vi "sendOutputData.vi"(8 "error in (no error)":errorcluster, 11 "Model in":refnum<class "Model.lvclass">) -> (0 "error out":errorcluster, 3 "Model out":refnum<class "Model.lvclass">)   [LabVIEW 2016, in "Model.lvclass"]
uses:
  Model.lvclass
  Typedefs/OutputData.ctl
  Model.lvclass/Model.ctl
  UserEvents/UserEvents.lvclass/UserEvents.ctl
  Common_ILC/ILC/ILC.lvclass/ILC.ctl
  ApplicationElements/Log/TestDataLog/TestDataLog.lvclass/TestDataLog.ctl
  Common_ILC/ILC/ILC.lvclass
  Typedefs/ILCBTTypedefs.lvlib
  UserEvents/UserEvents.lvclass
  ApplicationElements/Log/TestDataLog/TestDataLog.lvclass
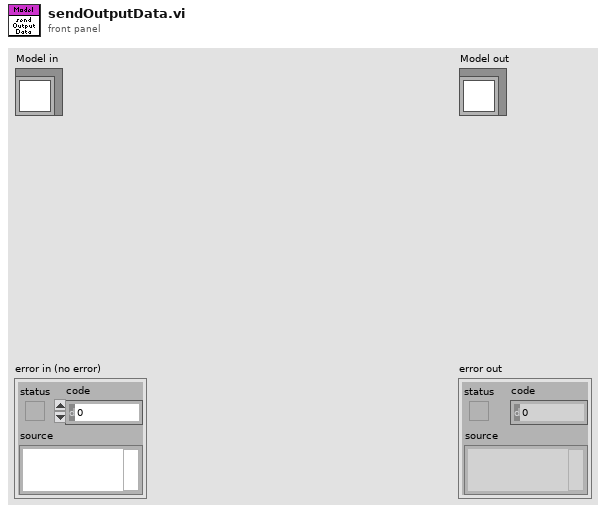
[diagram p1: front panel]
types:
  T1 = typedef "ILCBTTypedefs.lvlib/OutputData.ctl" = cluster{"Ch1":u16, "Ch2":u16, "Ch3":u16}
  T2 = typedef "ILCCommon.lvlib/ILCTypedefs.lvlib/Outputs.ctl" = cluster{"Step & Direction":i16, "Blower RPM":u8, "PWM (SSR)":u8, "Ch1":u16, "Ch2":u16, "Ch3":u16, "Ch4":u16}
  T3 = typedef "ILCBTTypedefs.lvlib/PubDataEvents.ctl" = cluster{"State":refnum<user-event>, "ErrorCode":refnum<user-event>, "OutputData":refnum<user-event>, "LogPath":refnum<user-event>, "TestScenarioCompleted":refnum<user-event>, "TestScenarioStarted":refnum<user-event>, "TestingStarted":refnum<user-event>, "StartTestScenario":refnum<user-event>}
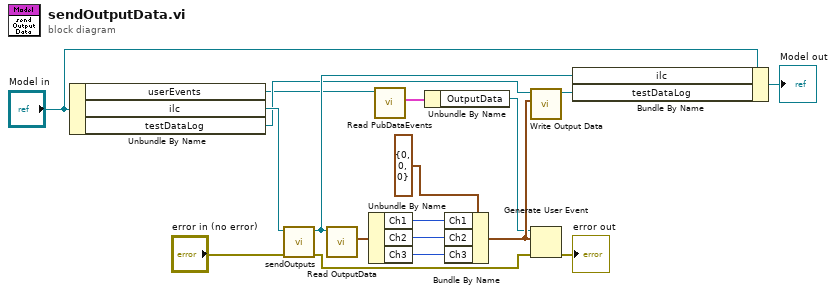
[diagram p0: block diagram]
diagram:
  n1 = Unbundle By Name("Model in") -> ("userEvents"=w4:refnum<class "UserEvents.lvclass">, "ilc"=w15:refnum<class "ILC.lvclass">, "testDataLog"=w8:refnum<class "TestDataLog.lvclass">)
  n2 = call "sendOutputs.vi"("error in (no error)"="error in (no error)", "ILC in"=w15) -> ("error out"=w3:errorcluster, "ILC out"=w13:refnum<class "ILC.lvclass">)  [unwired: 8 in]
  n3 = call "Read OutputData.vi"("ILC in"=w13) -> ("OutputData"=w11:T2)  [unwired: 9 in, 1 out]
  n4 = Unbundle By Name(w11) -> ("Ch1"=w10:u16, "Ch2"=w2:u16, "Ch3"=w1:u16)
  n5 = call "Read PubDataEvents.vi"("UserEvents in"=w4) -> ("PubDataEvents"=w6:T3)  [unwired: 9 in, 1 out]
  n6 = Unbundle By Name(w6) -> ("OutputData"=w5:refnum<user-event>)
  n7 = Bundle By Name(cluster=T1 {"Ch1"=0, "Ch2"=0, "Ch3"=0} ("event data"), "Ch1"=w10, "Ch2"=w2, "Ch3"=w1) -> (w9:T1)
  n8 = call "Write Output Data.vi"("Output Data"=w9, "TestDataLog in"=w8) -> ("TestDataLog out"=w7:refnum<class "TestDataLog.lvclass">)  [unwired: 9 in]
  n9 = Generate User Event(user event=w5, event data cluster=w9, error in=w3) -> (error out=→"error out":errorcluster)  [unwired: 1 in, 1 out]
  n10 = Bundle By Name(cluster="Model in", "ilc"=w13, "testDataLog"=w7) -> (→"Model out":refnum<class "Model.lvclass">)
